vi "rsscope_core_global.vi"() -> ()   [LabVIEW 2014] (continued)
the zoom area.\n\nAvailable Repeated Capabilities:\nNone\n\nRemote-control command(s):\nSEARch:RESDiagram:VERT:ABSolute:SPAN"}, {"Level"=3, "Class Only"=FALSE, "Identifier"="RSSCOPE_ATTR_SEARCH_RESULT_ZOOM_RELATIVE_VERTICAL_POSITION", "Descriptive Name"="Search Result Zoom Relative Vertical Position", "Data Type"=1, "Command"="SEAR:RESD:VERT:REL:POS", "Access"=2, "Range Table"="", "Read Callback"="rsscope_FormatSearchNameReal64_ReadCallback.vi", "Write Callback"="rsscope_FormatSearchNameReal64_WriteCallback.vi", "Supported Models"="", "Instrument Options"="", "Flags"=0, "Help"="Defines the y-value of the centerpoint of the zoom area.\n\nAvailable Repeated Capabilities:\nNone\n\nRemote-control command(s):\nSEARch:RESDiagram:VERT:RELative:POSition"}, {"Level"=3, "Class Only"=FALSE, "Identifier"="RSSCOPE_ATTR_SEARCH_RESULT_ZOOM_RELATIVE_VERTICAL_RANGE", "Descriptive Name"="Search Result Zoom Relative Vertical Range", "Data Type"=1, "Command"="SEAR:RESD:VERT:REL:SPAN", "Access"=2, "Range Table"="", "Read Callback"="rsscope_FormatSearchNameReal64_ReadCallback.vi", "Write Callback"="rsscope_FormatSearchNameReal64_WriteCallback.vi", "Supported Models"="", "Instrument Options"="", "Flags"=0, "Help"="Defines the width of the zoom area.\n\nAvailable Repeated Capabilities:\nNone\n\nRemote-control command(s):\nSEARch:RESDiagram:VERT:RELative:SPAN"}, {"Level"=2, "Class Only"=TRUE, "Identifier"="", "Descriptive Name"="Noise Reject", "Data Type"=0, "Command"="", "Access"=0, "Range Table"="", "Read Callback"="", "Write Callback"="", "Supported Models"="", "Instrument Options"="", "Flags"=0, "Help"="Noise rejection for searches is very similar to noise rejection for triggers. If the signal jitters inside this range and crosses the trigger level, no search result is detected."}, {"Level"=3, "Class Only"=FALSE, "Identifier"="RSSCOPE_ATTR_SEARCH_NOISE_REJECT_ENABLED", "Descriptive Name"="Search Noise Reject Enabled", "Data Type"=3, "Command"="SEAR:TRIG:LEV:NOIS", "Access"=2, "Range Table"="", "Read Callback"="rsscope_FormatSearchNameSourceBoolean_ReadCallback.vi", "Write Callback"="rsscope_FormatSearchNameSourceBoolean_WriteCallback.vi", "Supported Models"="", "Instrument Options"="", "Flags"=0, "Help"="If enabled, the noise reject settings for the waveform are considered for the search. Selected search name can be defined using RSSCOPE_ATTR_SELECTED_SEARCH_NAME, selected source can be defined using RSSCOPE_ATTR_SELECTED_SEARCH_SOURCE.\n\nAvailable Repeated Capabilities:\nNone\n\nRemote-control command(s):\nSEARch:TRIGger:LEVel:NOISe[:STATe]"}, {"Level"=3, "Class Only"=FALSE, "Identifier"="RSSCOPE_ATTR_SEARCH_NOISE_REJECT_HYSTERESIS_MODE", "Descriptive Name"="Search Noise Reject Hysteresis Mode", "Data Type"=0, "Command"="SEAR:TRIG:LEV:NOIS:MODE", "Access"=2, "Range Table"="rsscope_rngAbsRel", "Read Callback"="rsscope_FormatSearchNameSourceInt32_ReadCallback.vi", "Write Callback"="rsscope_FormatSearchNameSourceInt32_WriteCallback.vi", "Supported Models"="", "Instrument Options"="", "Flags"=0, "Help"="Defines whether absolute values or relative values to the vertical scaling are used as a hysteresis for noise rejection. Selected search name can be defined using RSSCOPE_ATTR_SELECTED_SEARCH_NAME, selected source can be defined using RSSCOPE_ATTR_SELECTED_SEARCH_SOURCE.\n\nAvailable Repeated Capabilities:\nNone\n\nRemote-control command(s):\nSEARch:TRIGger:LEVel:NOISe:MODE"}, {"Level"=3, "Class Only"=FALSE, "Identifier"="RSSCOPE_ATTR_SEARCH_NOISE_REJECT_ABSOLUTE_HYSTERESIS", "Descriptive Name"="Search Noise Reject Absolute Hysteresis", "Data Type"=1, "Command"="SEAR:TRIG:LEV:NOIS:ABS", "Access"=2, "Range Table"="", "Read Callback"="rsscope_FormatSearchNameSourceReal64_ReadCallback.vi", "Write Callback"="rsscope_FormatSearchNameSourceReal64_WriteCallback.vi", "Supported Models"="", "Instrument Options"="", "Flags"=0, "Help"="Defines the trigger hysteresis, a range in absolute values around the trigger level. If the signal jitters inside this range and crosses the trigger level, no trigger event is detected. Selected search name can be defined using RSSCOPE_ATTR_SELECTED_SEARCH_NAME, selected source can be defined using RSSCOPE_ATTR_SELECTED_SEARCH_SOURCE.\n\nAvailable Repeated Capabilities:\nNone\n\nRemote-control command(s):\nSEARch:TRIGger:LEVel:NOISe:ABSolute"}, {"Level"=3, "Class Only"=FALSE, "Identifier"="RSSCOPE_ATTR_SEARCH_NOISE_REJECT_RELATIVE_HYSTERESIS", "Descriptive Name"="Search Noise Reject Relative Hysteresis", "Data Type"=1, "Command"="SEAR:TRIG:LEV:NOIS:REL", "Access"=2, "Range Table"="RsScope_rngSearchNoiseRejectRelativeHysteresis", "Read Callback"="rsscope_FormatSearchNameSourceReal64_ReadCallback.vi", "Write Callback"="rsscope_FormatSearchNameSourceReal64_WriteCallback.vi", "Supported Models"="", "Instrument Options"="", "Flags"=0, "Help"="Defines a range around the trigger level in relative values. If the signal jitters inside this range and crosses the trigger level, no trigger event is detected. Selected search name can be defined using RSSCOPE_ATTR_SELECTED_SEARCH_NAME, selected source can be defined using RSSCOPE_ATTR_SELECTED_SEARCH_SOURCE.\n\nAvailable Repeated Capabilities:\nNone\n\nRemote-control command(s):\nSEARch:TRIGger:LEVel:NOISe:RELative"}, {"Level"=2, "Class Only"=TRUE, "Identifier"="", "Descriptive Name"="Serial Bus", "Data Type"=0, "Command"="", "Access"=0, "Range Table"="", "Read Callback"="", "Write Callback"="", "Supported Models"="", "Instrument Options"="", "Flags"=0, "Help"="Using the search functionality, you can find various events in the decoded data, the same events which you also can trigger on. Before you can start the search, you have to configure the bus correctly and acquire decoded data. To search on decoded data, set the search source to &apos;SerBus&apos; for the configured protocol."}, {"Level"=3, "Class Only"=TRUE, "Identifier"="", "Descriptive Name"="I2C", "Data Type"=0, "Command"="", "Access"=0, "Range Table"="", "Read Callback"="", "Write Callback"="", "Supported Models"="", "Instrument Options"="", "Flags"=0, "Help"="Configures I2C search settings."}, {"Level"=4, "Class Only"=FALSE, "Identifier"="RSSCOPE_ATTR_SEARCH_I2C_MODE", "Descriptive Name"="Search I2C Mode", "Data Type"=0, "Command"="SEAR:TRIG:I2C:MODE", "Access"=2, "Range Table"="rsscope_rngProtocolI2CTriggerType", "Read Callback"="rsscope_FormatSearchNameInt32_ReadCallback.vi", "Write Callback"="rsscope_FormatSearchNameInt32_WriteCallback.vi", "Supported Models"="", "Instrument Options"="K1", "Flags"=0, "Help"="Selects the search type for I2C analysis.\n\nAvailable Repeated Capabilities:\nNone\n\nRemote-control command(s):\nSEARch:TRIGger:I2C:MODE"}, {"Level"=4, "Class Only"=FALSE, "Identifier"="RSSCOPE_ATTR_SEARCH_I2C_CRITERIA_START", "Descriptive Name"="Search I2C Criteria Start", "Data Type"=3, "Command"="SEAR:TRIG:I2C:SCON", "Access"=2, "Range Table"="", "Read Callback"="rsscope_FormatSearchNameBoolean_ReadCallback.vi", "Write Callback"="rsscope_FormatSearchNameBoolean_WriteCallback.vi", "Supported Models"="", "Instrument Options"="K1", "Flags"=0, "Help"="Enables the search for the start of the message.\n\nAvailable Repeated Capabilities:\nNone\n\nRemote-control command(s):\nSEARch:TRIGger:I2C:SCONdition"}, {"Level"=4, "Class Only"=FALSE, "Identifier"="RSSCOPE_ATTR_SEARCH_I2C_CRITERIA_REPEATED_START", "Descriptive Name"="Search I2C Criteria Repeated Start", "Data Type"=3, "Command"="SEAR:TRIG:I2C:RCON", "Access"=2, "Range Table"="", "Read Callback"="rsscope_FormatSearchNameBoolean_ReadCallback.vi", "Write Callback"="rsscope_FormatSearchNameBoolean_WriteCallback.vi", "Supported Models"="", "Instrument Options"="K1", "Flags"=0, "Help"="Enables the search for a start condition without previous stop condition.\n\nAvailable Repeated Capabilities:\nNone\n\nRemote-control command(s):\nSEARch:TRIGger:I2C:RCONdition"}, {"Level"=4, "Class Only"=FALSE, "Identifier"="RSSCOPE_ATTR_SEARCH_I2C_CRITERIA_STOP", "Descriptive Name"="Search I2C Criteria Stop", "Data Type"=3, "Command"="SEAR:TRIG:I2C:STCN", "Access"=2, "Range Table"="", "Read Callback"="rsscope_FormatSearchNameBoolean_ReadCallback.vi", "Write Callback"="rsscope_FormatSearchNameBoolean_WriteCallback.vi", "Supported Models"="", "Instrument Options"="K1", "Flags"=0, "Help"="Enables the search for the start of the message.\n\nAvailable Repeated Capabilities:\nNone\n\nRemote-control command(s):\nSEARch:TRIGger:I2C:STCNdition"}, {"Level"=4, "Class Only"=FALSE, "Identifier"="RSSCOPE_ATTR_SEARCH_I2C_CRITERIA_NACK", "Descriptive Name"="Search I2C Criteria Nack", "Data Type"=3, "Command"="SEAR:TRIG:I2C:NACK", "Access"=2, "Range Table"="", "Read Callback"="rsscope_FormatSearchNameBoolean_ReadCallback.vi", "Write Callback"="rsscope_FormatSearchNameBoolean_WriteCallback.vi", "Supported Models"="", "Instrument Options"="K1", "Flags"=0, "Help"="Searches for missing address acknowledge bits.\n\nAvailable Repeated Capabilities:\nNone\n\nRemote-control command(s):\nSEARch:TRIGger:I2C:NACKnowledge"}, {"Level"=4, "Class Only"=FALSE, "Identifier"="RSSCOPE_ATTR_SEARCH_I2C_CRITERIA_ADDRESS", "Descriptive Name"="Search I2C Criteria Address", "Data Type"=3, "Command"="SEAR:TRIG:I2C:SADD", "Access"=2, "Range Table"="", "Read Callback"="rsscope_FormatSearchNameBoolean_ReadCallback.vi", "Write Callback"="rsscope_FormatSearchNameBoolean_WriteCallback.vi", "Supported Models"="", "Instrument Options"="K1", "Flags"=0, "Help"="Enables the search for one specific address condition or for a combination of address conditions.\n\nAvailable Repeated Capabilities:\nNone\n\nRemote-control command(s):\nSEARch:TRIGger:I2C:SADDress"}, {"Level"=4, "Class Only"=FALSE, "Identifier"="RSSCOPE_ATTR_SEARCH_I2C_CRITERIA_ADDRESS_OR", "Descriptive Name"="Search I2C Criteria Address OR", "Data Type"=3, "Command"="SEAR:TRIG:I2C:ADOR", "Access"=2, "Range Table"="", "Read Callback"="rsscope_FormatSearchNameBoolean_ReadCallback.vi", "Write Callback"="rsscope_FormatSearchNameBoolean_WriteCallback.vi", "Supported Models"="", "Instrument Options"="K1", "Flags"=0, "Help"="Enables the search for one to four address conditions.\n\nAvailable Repeated Capabilities:\nNone\n\nRemote-control command(s):\nSEARch:TRIGger:I2C:ADOR"}, {"Level"=4, "Class Only"=FALSE, "Identifier"="RSSCOPE_ATTR_SEARCH_I2C_CRITERIA_ADDRESS_DATA", "Descriptive Name"="Search I2C Criteria Address Data", "Data Type"=3, "Command"="SEAR:TRIG:I2C:ADD", "Access"=2, "Range Table"="", "Read Callback"="rsscope_FormatSearchNameBoolean_ReadCallback.vi", "Write Callback"="rsscope_FormatSearchNameBoolean_WriteCallback.vi", "Supported Models"="", "Instrument Options"="K1", "Flags"=0, "Help"="Enables the search for a combination of address and data conditions.\n\nAvailable Repeated Capabilities:\nNone\n\nRemote-control command(s):\nSEARch:TRIGger:I2C:ADData"}, {"Level"=4, "Class Only"=FALSE, "Identifier"="RSSCOPE_ATTR_SEARCH_I2C_ADRESS_NACK", "Descriptive Name"="Search I2C Adress Nack", "Data Type"=3, "Command"="SEAR:TRIG:I2C:ADN", "Access"=2, "Range Table"="", "Read Callback"="rsscope_FormatSearchNameBoolean_ReadCallback.vi", "Write Callback"="rsscope_FormatSearchNameBoolean_WriteCallback.vi", "Supported Models"="", "Instrument Options"="K1", "Flags"=0, "Help"="Searches if the address acknowledge bit is missing - no slave recognizes the address.\n\nAvailable Repeated Capabilities:\nNone\n\nRemote-control command(s):\nSEARch:TRIGger:I2C:ADNack"}, {"Level"=4, "Class Only"=FALSE, "Identifier"="RSSCOPE_ATTR_SEARCH_I2C_DATA_WRITE_NACK", "Descriptive Name"="Search I2C Data Write Nack", "Data Type"=3, "Command"="SEAR:TRIG:I2C:DWN", "Access"=2, "Range Table"="", "Read Callback"="rsscope_FormatSearchNameBoolean_ReadCallback.vi", "Write Callback"="rsscope_FormatSearchNameBoolean_WriteCallback.vi", "Supported Models"="", "Instrument Options"="K1", "Flags"=0, "Help"="Searches if a date acknowledge bit is missing - the addressed slave does not accept the data.\n\nAvailable Repeated Capabilities:\nNone\n\nRemote-control command(s):\nSEARch:TRIGger:I2C:DWNack"}, {"Level"=4, "Class Only"=FALSE, "Identifier"="RSSCOPE_ATTR_SEARCH_I2C_DATA_READ_NACK", "Descriptive Name"="Search I2C Data Read Nack", "Data Type"=3, "Command"="SEAR:TRIG:I2C:DRN", "Access"=2, "Range Table"="", "Read Callback"="rsscope_FormatSearchNameBoolean_ReadCallback.vi", "Write Callback"="rsscope_FormatSearchNameBoolean_WriteCallback.vi", "Supported Models"="", "Instrument Options"="K1", "Flags"=0, "Help"="Searches for the end of the read process when the master reads data from the slave. This Nack is sent according to the protocol definition, it is not an error.\n\nAvailable Repeated Capabilities:\nNone\n\nRemote-control command(s):\nSEARch:TRIGger:I2C:DRNack"}, {"Level"=4, "Class Only"=FALSE, "Identifier"="RSSCOPE_ATTR_SEARCH_I2C_ACCESS_BIT", "Descriptive Name"="Search I2C Access Bit", "Data Type"=0, "Command"="SEAR:TRIG:I2C:ACC", "Access"=2, "Range Table"="rsscope_rngProtocolI2CAccessBit", "Read Callback"="rsscope_FormatSearchNameInt32_ReadCallback.vi", "Write Callback"="rsscope_FormatSearchNameInt32_WriteCallback.vi", "Supported Models"="", "Instrument Options"="K1", "Flags"=0, "Help"="Sets the transfer direction of the data.\n\nAvailable Repeated Capabilities:\nNone\n\nRemote-control command(s):\nSEARch:TRIGger:I2C:ACCess"}, {"Level"=4, "Class Only"=FALSE, "Identifier"="RSSCOPE_ATTR_SEARCH_I2C_ADDRESS_TYPE", "Descriptive Name"="Search I2C Address Type", "Data Type"=0, "Command"="SEAR:TRIG:I2C:AMOD", "Access"=2, "Range Table"="rsscope_rngProtocolI2CAddressType", "Read Callback"="rsscope_FormatSearchNameInt32_ReadCallback.vi", "Write Callback"="rsscope_FormatSearchNameInt32_WriteCallback.vi", "Supported Models"="", "Instrument Options"="K1", "Flags"=0, "Help"="Sets the address length.\n\nAvailable Repeated Capabilities:\nNone\n\nRemote-control command(s):\nSEARch:TRIGger:I2C:AMODe"}, {"Level"=4, "Class Only"=FALSE, "Identifier"="RSSCOPE_ATTR_SEARCH_I2C_ADDRESS_CONDITION", "Descriptive Name"="Search I2C Address Condition", "Data Type"=0, "Command"="SEAR:TRIG:I2C:ACON", "Access"=2, "Range Table"="rsscope_rngProtocolTriggerCondition", "Read Callback"="rsscope_FormatSearchNameInt32_ReadCallback.vi", "Write Callback"="rsscope_FormatSearchNameInt32_WriteCallback.vi", "Supported Models"="", "Instrument Options"="K1", "Flags"=0, "Help"="Sets the operator to set a specific address or an address range.\n\nAvailable Repeated Capabilities:\nNone\n\nRemote-control command(s):\nSEARch:TRIGger:I2C:ACONdition"}, {"Level"=4, "Class Only"=FALSE, "Identifier"="RSSCOPE_ATTR_SEARCH_I2C_ADDRESS_MIN", "Descriptive Name"="Search I2C Address Min", "Data Type"=2, "Command"="SEAR:TRIG:I2C:ADDR", "Access"=2, "Range Table"="", "Read Callback"="rsscope_FormatSearchNameString_ReadCallback.vi", "Write Callback"="rsscope_FormatSearchNameString_WriteCallback.vi", "Supported Models"="", "Instrument Options"="K1", "Flags"=0, "Help"="Searches on the specified slave address, or sets the start value of an address range.\n\nValid Values: \nBinary pattern string consisting 1; 0; or X (any bit).\n\nAvailable Repeated Capabilities:\nNone\n\nRemote-control command(s):\nSEARch:TRIGger:I2C:ADDRess"}, {"Level"=4, "Class Only"=FALSE, "Identifier"="RSSCOPE_ATTR_SEARCH_I2C_ADDRESS_MAX", "Descriptive Name"="Search I2C Address Max", "Data Type"=2, "Command"="SEAR:TRIG:I2C:ADDT", "Access"=2, "Range Table"="", "Read Callback"="rsscope_FormatSearchNameString_ReadCallback.vi", "Write Callback"="rsscope_FormatSearchNameString_WriteCallback.vi", "Supported Models"="", "Instrument Options"="K1", "Flags"=0, "Help"="Sets the end value of an address range.\n\nValid Values: \nBinary pattern string consisting 1 and 0.\n\nAvailable Repeated Capabilities:\nNone\n\nRemote-control command(s):\nSEARch:TRIGger:I2C:ADDTo"}, {"Level"=4, "Class Only"=FALSE, "Identifier"="RSSCOPE_ATTR_SEARCH_I2C_POSITION_CONDITION", "Descriptive Name"="Search I2C Position Condition", "Data Type"=0, "Command"="SEAR:TRIG:I2C:DPOP", "Access"=2, "Range Table"="rsscope_rngI2CPositionCondition", "Read Callback"="rsscope_FormatSearchNameInt32_ReadCallback.vi", "Write Callback"="rsscope_FormatSearchNameInt32_WriteCallback.vi", "Supported Models"="", "Instrument Options"="K1", "Flags"=0, "Help"="Sets the operator for the data position.\n\nAvailable Repeated Capabilities:\nNone\n\nRemote-control command(s):\nSEARch:TRIGger:I2C:DPOPerator"}, {"Level"=4, "Class Only"=FALSE, "Identifier"="RSSCOPE_ATTR_SEARCH_I2C_POSITION_MIN", "Descriptive Name"="Search I2C Position Min", "Data Type"=0, "Command"="SEAR:TRIG:I2C:DPOS", "Access"=2, "Range Table"="rsscope_rnglI2CPositionMinMax", "Read Callback"="rsscope_FormatSearchNameInt32_ReadCallback.vi", "Write Callback"="rsscope_FormatSearchNameInt32_WriteCallback.vi", "Supported Models"="", "Instrument Options"="K1", "Flags"=0, "Help"="Sets the number of data bytes before the first byte of interest. These bytes are ignored.\n\nAvailable Repeated Capabilities:\nNone\n\nRemote-control command(s):\nSEARch:TRIGger:I2C:DPOSition"}, {"Level"=4, "Class Only"=FALSE, "Identifier"="RSSCOPE_ATTR_SEARCH_I2C_POSITION_MAX", "Descriptive Name"="Search I2C Position Max", "Data Type"=0, "Command"="SEAR:TRIG:I2C:DPTO", "Access"=2, "Range Table"="rsscope_rnglI2CPositionMinMax", "Read Callback"="rsscope_FormatSearchNameInt32_ReadCallback.vi", "Write Callback"="rsscope_FormatSearchNameInt32_WriteCallback.vi", "Supported Models"="", "Instrument Options"="K1", "Flags"=0, "Help"="Defines the last byte of interest.\n\nAvailable Repeated Capabilities:\nNone\n\nRemote-control command(s):\nSEARch:TRIGger:I2C:DPTO"}, {"Level"=4, "Class Only"=FALSE, "Identifier"="RSSCOPE_ATTR_SEARCH_I2C_DATA_CONDITION", "Descriptive Name"="Search I2C Data Condition", "Data Type"=0, "Command"="SEAR:TRIG:I2C:DCON", "Access"=2, "Range Table"="rsscope_rngProtocolTriggerCondition", "Read Callback"="rsscope_FormatSearchNameInt32_ReadCallback.vi", "Write Callback"="rsscope_FormatSearchNameInt32_WriteCallback.vi", "Supported Models"="", "Instrument Options"="K1", "Flags"=0, "Help"="Sets the operator to set a specific address or an address range.\n\nAvailable Repeated Capabilities:\nNone\n\nRemote-control command(s):\nSEARch:TRIGger:I2C:DCONdition"}, {"Level"=4, "Class Only"=FALSE, "Identifier"="RSSCOPE_ATTR_SEARCH_I2C_PATTERN_MIN", "Descriptive Name"="Search I2C Pattern Min", "Data Type"=2, "Command"="SEAR:TRIG:I2C:DMIN", "Access"=2, "Range Table"="", "Read Callback"="rsscope_FormatSearchNameString_ReadCallback.vi", "Write Callback"="rsscope_FormatSearchNameString_WriteCallback.vi", "Supported Models"="", "Instrument Options"="K1", "Flags"=0, "Help"="Specifies the data bit pattern, or sets the start value of a data pattern range. Enter the bytes in msb first bit order. The maximum pattern length is 64 bit. Waveform data is compared with the pattern byte-by-byte.\n\nAvailable Repeated Capabilities:\nNone\n\nRemote-control command(s):\nSEARch:TRIGger:I2C:DMIN"}, {"Level"=4, "Class Only"=FALSE, "Identifier"="RSSCOPE_ATTR_SEARCH_I2C_PATTERN_MAX", "Descriptive Name"="Search I2C Pattern Max", "Data Type"=2, "Command"="SEAR:TRIG:I2C:DMAX", "Access"=2, "Range Table"="", "Read Callback"="rsscope_FormatSearchNameString_ReadCallback.vi", "Write Callback"="rsscope_FormatSearchNameString_WriteCallback.vi", "Supported Models"="", "Instrument Options"="K1", "Flags"=0, "Help"="Sets the end value of an data range.\n\nAvailable Repeated Capabilities:\nNone\n\nRemote-control command(s):\nSEARch:TRIGger:I2C:DMAX"}, {"Level"=4, "Class Only"=TRUE, "Identifier"="", "Descriptive Name"="OR Slot", "Data Type"=0, "Command"="", "Access"=0, "Range Table"="", "Read Callback"="", "Write Callback"="", "Supported Models"="", "Instrument Options"="", "Flags"=0, "Help"="Index of the address in an &apos;address OR&apos; condition (OR slot)"}, {"Level"=5, "Class Only"=FALSE, "Identifier"="RSSCOPE_ATTR_SEARCH_I2C_ADDRESS_OR_STATE", "Descriptive Name"="Search I2C Address OR State", "Data Type"=3, "Command"="SEAR:TRIG:I2C:ADDO{ORSlot}:ENAB", "Access"=2, "Range Table"="", "Read Callback"="rsscope_FormatSearchNameBoolean_ReadCallback.vi", "Write Callback"="rsscope_FormatSearchNameBoolean_WriteCallback.vi", "Supported Models"="", "Instrument Options"="K1", "Flags"=0, "Help"="This attribute sets the state of the selected address OR slot for the &apos;address OR&apos; trigger condition\n\nAvailable Repeated Capabilities:\nORSlot: ORSlot1, ORSlot2, ORSlot3, ORSlot4\r\n\nRemote-control command(s):\nSEARch:TRIGger:I2C:ADDO<m>:ENABle"}, {"Level"=5, "Class Only"=FALSE, "Identifier"="RSSCOPE_ATTR_SEARCH_I2C_ADDRESS_OR_TYPE", "Descriptive Name"="Search I2C Address OR Type", "Data Type"=0, "Command"="SEAR:TRIG:I2C:ADDO{ORSlot}:ADRT", "Access"=2, "Range Table"="rsscope_rngProtocolI2CAddressORType", "Read Callback"="rsscope_FormatSearchNameInt32_ReadCallback.vi", "Write Callback"="rsscope_FormatSearchNameInt32_WriteCallback.vi", "Supported Models"="", "Instrument Options"="K1", "Flags"=0, "Help"="This attribute select address length.\n\nAvailable Repeated Capabilities:\nORSlot: ORSlot1, ORSlot2, ORSlot3, ORSlot4\r\n\nRemote-control command(s):\nSEARch:TRIGger:I2C:ADDO<m>:ADRType"}, {"Level"=5, "Class Only"=FALSE, "Identifier"="RSSCOPE_ATTR_SEARCH_I2C_ADDRESS_OR_ACCESS_BIT", "Descriptive Name"="Search I2C Address OR Access Bit", "Data Type"=0, "Command"="SEAR:TRIG:I2C:ADDO{ORSlot}:RWB", "Access"=2, "Range Table"="rsscope_rngProtocolI2CAccessBit", "Read Callback"="rsscope_FormatSearchNameInt32_ReadCallback.vi", "Write Callback"="rsscope_FormatSearchNameInt32_WriteCallback.vi", "Supported Models"="", "Instrument Options"="K1", "Flags"=0, "Help"="Sets the R/W bit of the indicated ADOR address in the &apos;address OR&apos; trigger condition.\n\nAvailable Repeated Capabilities:\nORSlot: ORSlot1, ORSlot2, ORSlot3, ORSlot4\r\n\nRemote-control command(s):\nSEARch:TRIGger:I2C:ADDO<m>:RWBit"}, {"Level"=5, "Class Only"=FALSE, "Identifier"="RSSCOPE_ATTR_SEARCH_I2C_ADDRESS_OR", "Descriptive Name"="Search I2C Address OR", "Data Type"=2, "Command"="SEAR:TRIG:I2C:ADDO{ORSlot}", "Access"=2, "Range Table"="", "Read Callback"="rsscope_FormatSearchNameString_ReadCallback.vi", "Write Callback"="rsscope_FormatSearchNameString_WriteCallback.vi", "Supported Models"="", "Instrument Options"="K1", "Flags"=0, "Help"="Sets the address pattern of the address.\n\nValid Values: \nBinary pattern string consisting 1; 0; or X (any bit).\n\nAvailable Repeated Capabilities:\nORSlot: ORSlot1, ORSlot2, ORSlot3, ORSlot4\r\n\nRemote-control command(s):\nSEARch:TRIGger:I2C:ADDO<m>[:VALue]"}, {"Level"=4, "Class Only"=TRUE, "Identifier"="", "Descriptive Name"="Results", "Data Type"=0, "Command"="", "Access"=0, "Range Table"="", "Read Callback"="", "Write Callback"="", "Supported Models"="", "Instrument Options"="", "Flags"=0, "Help"="Returns the search result of the specified frame."}, {"Level"=5, "Class Only"=FALSE, "Identifier"="RSSCOPE_ATTR_SEARCH_I2C_FRAME_COUNT", "Descriptive Name"="Search I2C Frame Count", "Data Type"=0, "Command"="SEAR:RES:I2C:FCO?", "Access"=0, "Range Table"="", "Read Callback"="rsscope_FormatSearchNameInt32_ReadCallback.vi", "Write Callback"="", "Supported Models"="", "Instrument Options"="K1", "Flags"=0, "Help"="Returns the frame count for the selected serial bus.\n\nAvailable Repeated Capabilities:\nNone\n\nRemote-control command(s):\nSEARch:RESult:I2C:FCOunt?"}, {"Level"=3, "Class Only"=TRUE, "Identifier"="", "Descriptive Name"="LIN", "Data Type"=0, "Command"="", "Access"=0, "Range Table"="", "Read Callback"="", "Write Callback"="", "Supported Models"="", "Instrument Options"="", "Flags"=0, "Help"="Configures LIN search settings."}, {"Level"=4, "Class Only"=FALSE, "Identifier"="RSSCOPE_ATTR_SEARCH_LIN_MODE", "Descriptive Name"="Search LIN Mode", "Data Type"=0, "Command"="SEAR:TRIG:LIN:TYPE", "Access"=2, "Range Table"="rsscope_rngProtocolLINTrigger", "Read Callback"="rsscope_FormatSearchNameInt32_ReadCallback.vi", "Write Callback"="rsscope_FormatSearchNameInt32_WriteCallback.vi", "Supported Models"="", "Instrument Options"="K0|K3", "Flags"=0, "Help"="Selects the search type for LIN analysis.\n\nAvailable Repeated Capabilities:\nNone\n\nRemote-control command(s):\nSEARch:TRIGger:LIN:TYPE"}, {"Level"=4, "Class Only"=TRUE, "Identifier"="", "Descriptive Name"="Criteria", "Data Type"=0, "Command"="", "Access"=0, "Range Table"="", "Read Callback"="", "Write Callback"="", "Supported Models"="", "Instrument Options"="", "Flags"=0, "Help"="Configures search criteria."}, {"Level"=5, "Class Only"=FALSE, "Identifier"="RSSCOPE_ATTR_SEARCH_LIN_CRITERIA_START_OF_FRAME", "Descriptive Name"="Search LIN Criteria Start Of Frame", "Data Type"=3, "Command"="SEAR:TRIG:LIN:SSOF", "Access"=2, "Range Table"="", "Read Callback"="rsscope_FormatSearchNameBoolean_ReadCallback.vi", "Write Callback"="rsscope_FormatSearchNameBoolean_WriteCallback.vi", "Supported Models"="", "Instrument Options"="K3", "Flags"=0, "Help"="Enables the search for the stop bit of the sync field, which marks the frame start.\n\nAvailable Repeated Capabilities:\nNone\n\nRemote-control command(s):\nSEARch:TRIGger:LIN:SSOFrame"}, {"Level"=5, "Class Only"=FALSE, "Identifier"="RSSCOPE_ATTR_SEARCH_LIN_CRITERIA_IDENTIFIER", "Descriptive Name"="Search LIN Criteria Identifier", "Data Type"=3, "Command"="SEAR:TRIG:LIN:SFID", "Access"=2, "Range Table"="", "Read Callback"="rsscope_FormatSearchNameBoolean_ReadCallback.vi", "Write Callback"="rsscope_FormatSearchNameBoolean_WriteCallback.vi", "Supported Models"="", "Instrument Options"="K3", "Flags"=0, "Help"="Enables the search for one specific identifier or an identifier range.\n\nAvailable Repeated Capabilities:\nNone\n\nRemote-control command(s):\nSEARch:TRIGger:LIN:SFIDentifier"}, {"Level"=5, "Class Only"=FALSE, "Identifier"="RSSCOPE_ATTR_SEARCH_LIN_CRITERIA_IDENTIFIER_OR", "Descriptive Name"="Search LIN Criteria Identifier OR", "Data Type"=3, "Command"="SEAR:TRIG:LIN:IDEN", "Access"=2, "Range Table"="", "Read Callback"="rsscope_FormatSearchNameBoolean_ReadCallback.vi", "Write Callback"="rsscope_FormatSearchNameBoolean_WriteCallback.vi", "Supported Models"="", "Instrument Options"="K3", "Flags"=0, "Help"="Enables the search for one to four address conditions.\n\nAvailable Repeated Capabilities:\nNone\n\nRemote-control command(s):\nSEARch:TRIGger:LIN:IDENtifieror"}, {"Level"=5, "Class Only"=FALSE, "Identifier"="RSSCOPE_ATTR_SEARCH_LIN_CRITERIA_IDENTIFIER_DATA", "Descriptive Name"="Search LIN Criteria Identifier Data", "Data Type"=3, "Command"="SEAR:TRIG:LIN:SIDD", "Access"=2, "Range Table"="", "Read Callback"="rsscope_FormatSearchNameBoolean_ReadCallback.vi", "Write Callback"="rsscope_FormatSearchNameBoolean_WriteCallback.vi", "Supported Models"="", "Instrument Options"="K3", "Flags"=0, "Help"="Enables the search for a combination of identifier and data conditions.\n\nAvailable Repeated Capabilities:\nNone\n\nRemote-control command(s):\nSEARch:TRIGger:LIN:SIDData"}, {"Level"=5, "Class Only"=FALSE, "Identifier"="RSSCOPE_ATTR_SEARCH_LIN_CRITERIA_WAKEUP_FRAME", "Descriptive Name"="Search LIN Criteria Wakeup Frame", "Data Type"=3, "Command"="SEAR:TRIG:LIN:WUFR", "Access"=2, "Range Table"="", "Read Callback"="rsscope_FormatSearchNameBoolean_ReadCallback.vi", "Write Callback"="rsscope_FormatSearchNameBoolean_WriteCallback.vi", "Supported Models"="", "Instrument Options"="K3", "Flags"=0, "Help"="Enables the search for wakeup frames.\n\nAvailable Repeated Capabilities:\nNone\n\nRemote-control command(s):\nSEARch:TRIGger:LIN:WUFRame"}, {"Level"=5, "Class Only"=FALSE, "Identifier"="RSSCOPE_ATTR_SEARCH_LIN_CRITERIA_ERROR_CONDITION", "Descriptive Name"="Search LIN Criteria Error Condition", "Data Type"=3, "Command"="SEAR:TRIG:LIN:SERR", "Access"=2, "Range Table"="", "Read Callback"="rsscope_FormatSearchNameBoolean_ReadCallback.vi", "Write Callback"="rsscope_FormatSearchNameBoolean_WriteCallback.vi", "Supported Models"="", "Instrument Options"="K3", "Flags"=0, "Help"="Enables the search for various errors in the frame.\n\nAvailable Repeated Capabilities:\nNone\n\nRemote-control command(s):\nSEARch:TRIGger:LIN:SERRor"}, {"Level"=4, "Class Only"=TRUE, "Identifier"="", "Descriptive Name"="Data", "Data Type"=0, "Command"="", "Access"=0, "Range Table"="", "Read Callback"="", "Write Callback"="", "Supported Models"="", "Instrument Options"="", "Flags"=0, "Help"="Configures data setup."}, {"Level"=5, "Class Only"=FALSE, "Identifier"="RSSCOPE_ATTR_SEARCH_LIN_CONDITION_DATA", "Descriptive Name"="Search LIN Condition Data", "Data Type"=0, "Command"="SEAR:TRIG:LIN:DCON", "Access"=2, "Range Table"="rsscope_rngProtocolTriggerCondition", "Read Callback"="rsscope_FormatSearchNameInt32_ReadCallback.vi", "Write Callback"="rsscope_FormatSearchNameInt32_WriteCallback.vi", "Supported Models"="", "Instrument Options"="K3", "Flags"=0, "Help"="Sets the operator to set a specific data or an data range.\n\nAvailable Repeated Capabilities:\nNone\n\nRemote-control command(s):\nSEARch:TRIGger:LIN:DCONdition"}, {"Level"=5, "Class Only"=FALSE, "Identifier"="RSSCOPE_ATTR_SEARCH_LIN_PATTERN_DATA_MIN", "Descriptive Name"="Search LIN Pattern Data Min", "Data Type"=2, "Command"="SEAR:TRIG:LIN:DMIN", "Access"=2, "Range Table"="", "Read Callback"="rsscope_FormatSearchNameString_ReadCallback.vi", "Write Callback"="rsscope_FormatSearchNameString_WriteCallback.vi", "Supported Models"="", "Instrument Options"="K3", "Flags"=0, "Help"="Specifies a data pattern, or sets the start value of a data pattern range.\n\nNote(s):\n\n(1) Valid values 1; 0; or X (any bit), use of X is restricted to the conditions &apos;Equal&apos; and &apos;Not equal&apos;.\n\n(2) Data binary pattern string consist 8 Bytes.\n\nAvailable Repeated Capabilities:\nNone\n\nRemote-control command(s):\nSEARch:TRIGger:LIN:DMIN"}, {"Level"=5, "Class Only"=FALSE, "Identifier"="RSSCOPE_ATTR_SEARCH_LIN_PATTERN_DATA_MAX", "Descriptive Name"="Search LIN Pattern Data Max", "Data Type"=2, "Command"="SEAR:TRIG:LIN:DMAX", "Access"=2, "Range Table"="", "Read Callback"="rsscope_FormatSearchNameString_ReadCallback.vi", "Write Callback"="rsscope_FormatSearchNameString_WriteCallback.vi", "Supported Models"="", "Instrument Options"="K3", "Flags"=0, "Help"="Sets the end value of data pattern range if condition is &apos;In range&apos; and &apos;Out of range&apos;.\n \nNote(s):\n(1) Valid values 1; 0; or X (any bit), use of X is restricted to the conditions &apos;Equal&apos; and &apos;Not equal&apos;.\n\n(2) Data binary pattern string consist 8 Bytes.\n\nAvailable Repeated Capabilities:\nNone\n\nRemote-control command(s):\nSEARch:TRIGger:LIN:DMAX"}, {"Level"=5, "Class Only"=FALSE, "Identifier"="RSSCOPE_ATTR_SEARCH_LIN_DATA_LENGTH_CONDITION", "Descriptive Name"="Search LIN Data Length Condition", "Data Type"=0, "Command"="SEAR:TRIG:LIN:DLEC", "Access"=2, "Range Table"="rsscope_rngProtocolLINTriggerDataCondition", "Read Callback"="rsscope_FormatSearchNameInt32_ReadCallback.vi", "Write Callback"="rsscope_FormatSearchNameInt32_WriteCallback.vi", "Supported Models"="", "Instrument Options"="K3", "Flags"=0, "Help"="Sets the operator to set the data length code for triggering on LIN data. For big endian transfer direction, you can trigger on a number of bytes less than the data length of the frame, that means, on the beginning of the data pattern. For little endian transfer direction, the exact number of data bytes in the frame must be set.\n\nAvailable Repeated Capabilities:\nNone\n\nRemote-control command(s):\nSEARch:TRIGger:LIN:DLECondition"}, {"Level"=5, "Class Only"=FALSE, "Identifier"="RSSCOPE_ATTR_SEARCH_LIN_DATA_LENGTH", "Descriptive Name"="Search LIN Data Length", "Data Type"=0, "Command"="SEAR:TRIG:LIN:DLEN", "Access"=2, "Range Table"="rsscope_rngLINDataLength", "Read Callback"="rsscope_FormatSearchNameInt32_ReadCallback.vi", "Write Callback"="rsscope_FormatSearchNameInt32_WriteCallback.vi", "Supported Models"="", "Instrument Options"="K3", "Flags"=0, "Help"="Sets the length of the bit pattern to be found, in bytes. For &apos;Big Endian&apos; transfer direction, you can trigger on a number of bytes less than the data length of the frame, that means, on the beginning of the data pattern. For &apos;Little Endian&apos; transfer direction, the exact number of data bytes in the frame must be set.\n\nAvailable Repeated Capabilities:\nNone\n\nRemote-control command(s):\nSEARch:TRIGger:LIN:DLENgth"}, {"Level"=5, "Class Only"=FALSE, "Identifier"="RSSCOPE_ATTR_SEARCH_LIN_DATA_TRANSFER", "Descriptive Name"="Search LIN Data Transfer", "Data Type"=0, "Command"="SEAR:TRIG:LIN:BORD", "Access"=2, "Range Table"="rsscope_rngLINDataTransfer", "Read Callback"="rsscope_FormatSearchNameInt32_ReadCallback.vi", "Write Callback"="rsscope_FormatSearchNameInt32_WriteCallback.vi", "Supported Models"="", "Instrument Options"="K3", "Flags"=0, "Help"="Sets the byte order (endianness) of the data transfer.\n\nAvailable Repeated Capabilities:\nNone\n\nRemote-control command(s):\nSEARch:TRIGger:LIN:BORDer"}, {"Level"=4, "Class Only"=TRUE, "Identifier"="", "Descriptive Name"="Identifier", "Data Type"=0, "Command"="", "Access"=0, "Range Table"="", "Read Callback"="", "Write Callback"="", "Supported Models"="", "Instrument Options"="", "Flags"=0, "Help"="Configures identifier setup."}, {"Level"=5, "Class Only"=FALSE, "Identifier"="RSSCOPE_ATTR_SEARCH_LIN_IDENTIFIER_CONDITION", "Descriptive Name"="Search LIN Identifier Condition", "Data Type"=0, "Command"="SEAR:TRIG:LIN:ICON", "Access"=2, "Range Table"="rsscope_rngProtocolTriggerCondition", "Read Callback"="rsscope_FormatSearchNameInt32_ReadCallback.vi", "Write Callback"="rsscope_FormatSearchNameInt32_WriteCallback.vi", "Supported Models"="", "Instrument Options"="K3", "Flags"=0, "Help"="Sets the operator to set a specific identifier or an identifier range.\n\nAvailable Repeated Capabilities:\nNone\n\nRemote-control command(s):\nSEARch:TRIGger:LIN:ICONdition"}, {"Level"=5, "Class Only"=FALSE, "Identifier"="RSSCOPE_ATTR_SEARCH_LIN_PATTERN_IDENTIFIER_MIN", "Descriptive Name"="Search LIN Pattern Identifier Min", "Data Type"=2, "Command"="SEAR:TRIG:LIN:IMIN", "Access"=2, "Range Table"="", "Read Callback"="rsscope_FormatSearchNameString_ReadCallback.vi", "Write Callback"="rsscope_FormatSearchNameString_WriteCallback.vi", "Supported Models"="", "Instrument Options"="K3", "Flags"=0, "Help"="Specifies a slave identifier pattern, or sets the start value of an pattern range.\n\nNote(s):\n\n(1) Valid values 1; 0; or X (any bit), use of X is restricted to the conditions &apos;Equal&apos; and &apos;Not equal&apos;.\n\n(2) ID binary pattern string consist 6 bits.\n\nAvailable Repeated Capabilities:\nNone\n\nRemote-control command(s):\nSEARch:TRIGger:LIN:IMIN"}, {"Level"=5, "Class Only"=FALSE, "Identifier"="RSSCOPE_ATTR_SEARCH_LIN_PATTERN_IDENTIFIER_MAX", "Descriptive Name"="Search LIN Pattern Identifier Max", "Data Type"=2, "Command"="SEAR:TRIG:LIN:IMAX", "Access"=2, "Range Table"="", "Read Callback"="rsscope_FormatSearchNameString_ReadCallback.vi", "Write Callback"="rsscope_FormatSearchNameString_WriteCallback.vi", "Supported Models"="", "Instrument Options"="K3", "Flags"=0, "Help"="Sets the end value of an identifier range if condition is &apos;In range&apos; and &apos;Out of range&apos;.\n \nNote(s):\n(1) Valid values 1; 0; or X (any bit), use of X is restricted to the conditions &apos;Equal&apos; and &apos;Not equal&apos;.\n\n(2) ID binary pattern string consist 6 bits.\n\nAvailable Repeated Capabilities:\nNone\n\nRemote-control command(s):\nSEARch:TRIGger:LIN:IMAX"}, {"Level"=4, "Class Only"=TRUE, "Identifier"="", "Descriptive Name"="OR Slot", "Data Type"=0, "Command"="", "Access"=0, "Range Table"="", "Read Callback"="", "Write Callback"="", "Supported Models"="", "Instrument Options"="", "Flags"=0, "Help"="Sets the trigger to a combination of up to four identifiers. Enter the patterns in the &apos;Frame\nID&apos; fields. In binary and hex format, characters 1, 0, and X (don&apos;t care) are allowed. For\neach identifier pattern to be triggered on, enable &apos;Monitor&apos;."}, {"Level"=5, "Class Only"=FALSE, "Identifier"="RSSCOPE_ATTR_SEARCH_LIN_ADDRESS_OR_STATE", "Descriptive Name"="Search LIN Address OR State", "Data Type"=3, "Command"="SEAR:TRIG:LIN:IDOR{ORSlot}:ENAB", "Access"=2, "Range Table"="", "Read Callback"="rsscope_FormatSearchNameBoolean_ReadCallback.vi", "Write Callback"="rsscope_FormatSearchNameBoolean_WriteCallback.vi", "Supported Models"="", "Instrument Options"="K3", "Flags"=0, "Help"="Includes the indicated IDOR address in the &apos;identifier OR&apos; search.\n\nAvailable Repeated Capabilities:\nORSlot: ORSlot1, ORSlot2, ORSlot3, ORSlot4\r\n\nRemote-control command(s):\nSEARch:TRIGger:LIN:IDOR<m>:ENABle"}, {"Level"=5, "Class Only"=FALSE, "Identifier"="RSSCOPE_ATTR_SEARCH_LIN_ADDRESS_OR", "Descriptive Name"="Search LIN Address OR", "Data Type"=2, "Command"="SEAR:TRIG:LIN:IDOR{ORSlot}", "Access"=2, "Range Table"="", "Read Callback"="rsscope_FormatSearchNameString_ReadCallback.vi", "Write Callback"="rsscope_FormatSearchNameString_WriteCallback.vi", "Supported Models"="", "Instrument Options"="K3", "Flags"=0, "Help"="Defines the pattern of the indicated IDOR identifier in the &apos;identifier OR&apos; trigger condition.\n\nValid Values: \nBinary pattern string consisting bits of 1; 0; or X (any bit).\n\nAvailable Repeated Capabilities:\nORSlot: ORSlot1, ORSlot2, ORSlot3, ORSlot4\r\n\nRemote-control command(s):\nSEARch:TRIGger:LIN:IDOR<m>[:VALue]"}, {"Level"=4, "Class Only"=TRUE, "Identifier"="", "Descriptive Name"="Error Conditions", "Data Type"=0, "Command"="", "Access"=0, "Range Table"="", "Read Callback"="", "Write Callback"="", "Supported Models"="", "Instrument Options"="", "Flags"=0, "Help"="Triggers if one or more of the following errors occur: Checksum error, Identifier parity error, Sync error."}, {"Level"=5, "Class Only"=FALSE, "Identifier"="RSSCOPE_ATTR_SEARCH_LIN_CHECKSUM_ERROR", "Descriptive Name"="Search LIN Checksum Error", "Data Type"=3, "Command"="SEAR:TRIG:LIN:CHKS", "Access"=2, "Range Table"="", "Read Callback"="rsscope_FormatSearchNameBoolean_ReadCallback.vi", "Write Callback"="rsscope_FormatSearchNameBoolean_WriteCallback.vi", "Supported Models"="", "Instrument Options"="K3", "Flags"=0, "Help"="Searches for checksum errors according to the LIN standard.\n\nAvailable Repeated Capabilities:\nNone\n\nRemote-control command(s):\nSEARch:TRIGger:LIN:CHKSerror"}, {"Level"=5, "Class Only"=FALSE, "Identifier"="RSSCOPE_ATTR_SEARCH_LIN_CRC_ERROR_PATTERN", "Descriptive Name"="Search LIN CRC Error Pattern", "Data Type"=2, "Command"="SEAR:TRIG:LIN:ERRP", "Access"=2, "Range Table"="", "Read Callback"="rsscope_FormatSearchNameString_ReadCallback.vi", "Write Callback"="rsscope_FormatSearchNameString_WriteCallback.vi", "Supported Models"="", "Instrument Options"="K3", "Flags"=0, "Help"="Sets bit pattern of the slave identifier (&apos;ID&apos;).\n\nValid Values: \nBinary pattern string consisting 1; 0; or X (any bit).\n\nAvailable Repeated Capabilities:\nNone\n\nRemote-control command(s):\nSEARch:TRIGger:LIN:ERRPattern"}, {"Level"=5, "Class Only"=FALSE, "Identifier"="RSSCOPE_ATTR_SEARCH_LIN_CRC_ERROR_DATA_LENGTH", "Descriptive Name"="Search LIN CRC Error Data Length", "Data Type"=0, "Command"="SEAR:TRIG:LIN:CRCD", "Access"=2, "Range Table"="rsscope_rngLINTriggerCRCErrDataLength", "Read Callback"="rsscope_FormatSearchNameInt32_ReadCallback.vi", "Write Callback"="rsscope_FormatSearchNameInt32_WriteCallback.vi", "Supported Models"="", "Instrument Options"="K3", "Flags"=0, "Help"="Sets the number of data bytes search for CRC errors.\n\nAvailable Repeated Capabilities:\nNone\n\nRemote-control command(s):\nSEARch:TRIGger:LIN:CRCDatalen"}, {"Level"=5, "Class Only"=FALSE, "Identifier"="RSSCOPE_ATTR_SEARCH_LIN_CRC_STANDARD", "Descriptive Name"="Search LIN CRC Standard", "Data Type"=0, "Command"="SEAR:TRIG:LIN:STAN", "Access"=2, "Range Table"="rsscope_rngProtocolLINTriggerCRCStandard", "Read Callback"="rsscope_FormatSearchNameInt32_ReadCallback.vi", "Write Callback"="rsscope_FormatSearchNameInt32_WriteCallback.vi", "Supported
